vi "Symulowane dane z robota.vi"   [LabVIEW 2015, in "Biblioteka moduł map v3.lvlib" / "Generatory_symulatory.lvlib"]
uses:
  Generatory_symulatory.lvlib
  <vilib>/Platform/TimedLoop/XDataNode/timing_clust.ctl
  <vilib>/Platform/TimedLoop/XDataNode/nitl_modes.ctl
  <vilib>/Platform/TimedLoop/XDataNode/wakeup.ctl
  Zmienne/szablon odometry_filtered_local.ctl
  Zmienne/szablon odometry_filtered_local.vi
  <vilib>/platform/TimedLoop/XDataNode/XDataNode.xnode
  Zmienne/Zmienne.lvlib
  <vilib>/Platform/TimedLoop/XDataNode/XDNodeRunTimeDep.lvlib
types:
  T1 = typedef "Biblioteka moduł map v3.lvlib/Zmienne.lvlib/szablon odometry_filtered_local.ctl" = cluster{"topic":string, "msg":cluster{"header":cluster{"seq":u32, "stamp":cluster{"secs":u32, "nsecs":i32}, "frame_id":string}, "child_frame_id":string, "pose":cluster{"pose":cluster{"position":cluster{"y":dbl, "z":dbl, "x":dbl}, "orientation":cluster{"y":dbl, "z":dbl, "x":dbl, "w":dbl}}, "covariance":dbl[]}, "twist":cluster{"twist":cluster{"linear":cluster{"y":dbl, "z":dbl, "x":dbl}, "angular":cluster{"y":dbl, "z":dbl, "x":dbl}}, "covariance":dbl[]}}, "op":string}
  T2 = typedef "XDNodeRunTimeDep.lvlib/timing_clust.ctl" = cluster{"Expected End [f-1]":u64, "Actual End [f-1]":u64, "Finished Late? [f-1]":bool, "Expected End [i-1]":u64, "Actual End [i-1]":u64, "Finished Late? [i-1]":bool, "Expected Start [i]":u64, "Actual Start [i]":u64, "Expected Start [f]":u64, "Actual Start [f]":u64, "Source Name":string, "Structure Name":string, "Period":i64, "Deadline":i64, "Offset":i64, "Start":i64, "Priority":i32, "Timeout":i32, "Mode":T3, "Wakeup Reason":T4, "Error":errorcluster, "Source Type":string, "Secondary Source Type":string, "Global End Time":u64, "Global Start Time":u64, "Frame Duration":u64, "Iteration Duration":u64, "Assigned CPU":i32, "I/O Scan Engine Mode":u32}
  T3 = typedef "XDNodeRunTimeDep.lvlib/nitl_modes.ctl" = enum32{"No Change", "Process missed periods, maintain original phase", "Discard missed periods, maintain original phase", "Process missed periods, ignore original phase", "Discard missed periods, ignore original phase"}
  T4 = typedef "XDNodeRunTimeDep.lvlib/wakeup.ctl" = enum32{"Normal", "Aborted", "Asynchronous wakeup", "Timing source error", "Timed loop error", "Timeout"}
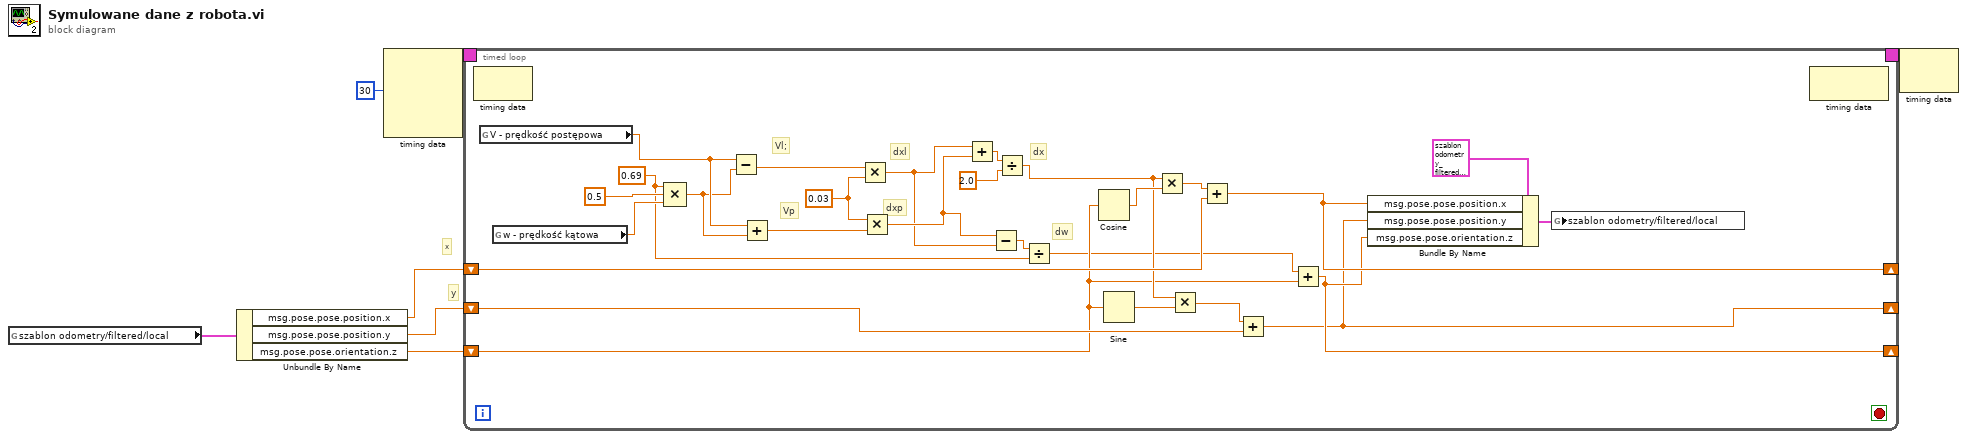
[diagram p0: block diagram]
diagram:
  # "y"
  # "x"
  n1 = global read "szablon odometry_filtered_local.vi" "szablon odometry/filtered/local"() -> (w4:T1)
  n2 = Unbundle By Name(w4) -> ("msg.pose.pose.position.x"=w2:dbl, "msg.pose.pose.position.y"=w1:dbl, "msg.pose.pose.orientation.z"=w3:dbl)
  n3 = node-c288(i64 30 ("Period")) -> (w7:T2)  [unwired: 3 in]
  n4 = timed-loop {
    timing: w7 -> [_]
    timing-out: [_] -> w6
    shift-right: [w9] -> _
    shift-left: w3 -> [w12]
    shift-right: [w8] -> _
    shift-left: w1 -> [w15]
    shift-right: [w10] -> _
    shift-left: w2 -> [w17]
    stop <- _ stop-if-true
    w26 = 0.03 ("y")
    w20 = 0.69 ("value")
    # "dw"
    # "dx"
    # "dxl"
    # "dxp"
    # "Vp"
    # "Vl;"
    n5 = node-c288() -> ()  [unwired: 1 in, 1 out]
    n6 = global read "V - prędkość postępowa.vi" "V - prędkość postępowa"() -> (w30:dbl)
    n7 = global read "w - prękdość kątowa.vi" "w - prędkość kątowa"() -> (w31:dbl)
    n8 = Compound Arithmetic op=MULTIPLY(w20, 0.5 ("value"), w31) -> (w29:dbl)
    n9 = Subtract(x=w30, y=w29) -> (x-y=w28:dbl)
    n10 = Add(x=w30, y=w29) -> (x+y=w27:dbl)
    n11 = Multiply(x=w28, y=w26) -> (x*y=w22:dbl)
    n12 = Multiply(x=w26, y=w27) -> (x*y=w23:dbl)
    n13 = Add(x=w22, y=w23) -> (x+y=w25:dbl)
    n14 = Subtract(x=w23, y=w22) -> (x-y=w21:dbl)
    n15 = Divide(x=w25, y=2.0) -> (x/y=w14:dbl)
    n16 = Divide(x=w21, y=w20) -> (x/y=w11:dbl)
    n17 = Cosine(x=w12) -> (cos(x)=w19:dbl)
    n18 = Sine(x=w12) -> (sin(x)=w13:dbl)
    n19 = Multiply(x=w14, y=w19) -> (x*y=w18:dbl)
    n20 = Multiply(x=w14, y=w13) -> (x*y=w16:dbl)
    n21 = Add(x=w18, y=w17) -> (x+y=w10:dbl)
    n22 = Add(x=w16, y=w15) -> (x+y=w8:dbl)
    n23 = Add(x=w11, y=w12) -> (x+y=w9:dbl)
    n24 = Bundle By Name(cluster=T1 {"topic"="", "msg"={"header"={"seq"=0, "stamp"={"secs"=0, "nsecs"=0}, "frame_id"=""}, "child_frame_id"="", "pose"={"pose"={"position"={"y"=0.0, "z"=0.0, "x"=0.0}, "orientation"={"y"=0.0, "z"=0.0, "x"=0.0, "w"=0.0}}, "covariance"=[]}, "twist"={"twist"={"linear"={"y"=0.0, "z"=0.0, "x"=0.0}, "angular"={"y"=0.0, "z"=0.0, "x"=0.0}}, "covariance"=[]}}, "op"=""} ("szablon odometry/filtered/local"), "msg.pose.pose.position.x"=w10, "msg.pose.pose.position.y"=w8, "msg.pose.pose.orientation.z"=w9) -> (w33:T1)
    n25 = global write "szablon odometry_filtered_local.vi" "szablon odometry/filtered/local"(w33) -> ()
    n26 = node-c288() -> ()  [unwired: 1 in, 1 out]
  }
  n27 = node-c288(w6) -> ()  [unwired: 1 out]
